vi "Get Transfer UIs.vi"(8 "error in (no error)":errorcluster, 11 "Component UI in":refnum<class "Component User Interfaces.lvclass">) -> (0 "error out":errorcluster, 1 "Tx Transfer UI":refnum<class "User Interface.lvclass">, 2 "Rx Transfer UI":refnum<class "User Interface.lvclass">, 3 "Component UI out":refnum<class "Component User Interfaces.lvclass">)   [LabVIEW 2020, in "DSF Core.lvlib" / "Component User Interfaces.lvclass"]
uses:
  Component User Interfaces.lvclass
  User Interface/User Interface.lvclass
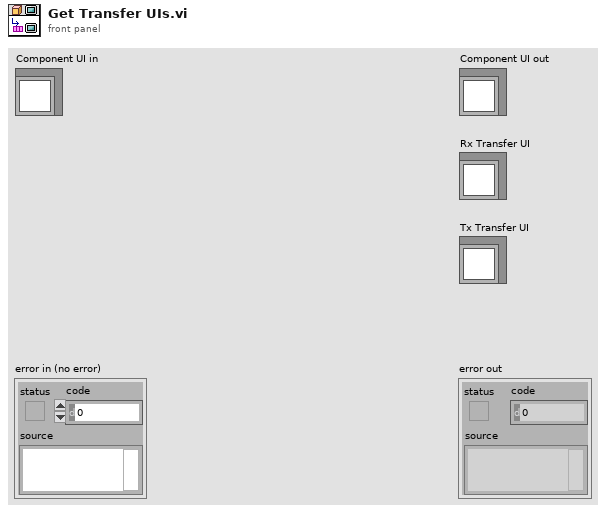
[diagram p1: front panel]
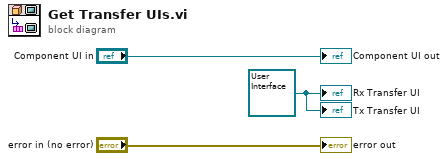
[diagram p0: block diagram]
diagram:
  w1 = refnum<class "User Interface.lvclass"> refnum ("Rx Transfer UI")
  "error out" <- "error in (no error)"
  "Component UI out" <- "Component UI in"
  "Rx Transfer UI" <- w1
  "Tx Transfer UI" <- w1
